vi "Escape_URL_method.vi"(8 "error in (no error)":errorcluster, 10 "Escape URLs?":bool, 11 "URL In":string) -> (0 "error out":errorcluster, 3 "URL Out":string)   [LabVIEW 2016]
uses:
  <vilib>/wsapi/NI_WebServices.lvlib
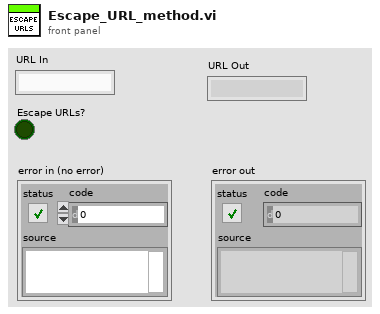
[diagram p1: front panel]
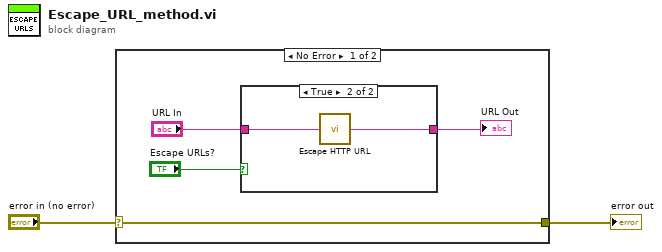
[diagram p0: block diagram]
diagram:
  n1 = case shown="No Error" "error in (no error)" {
    selector: "error in (no error)" -> [w3 w10]
    tunnel: [w3 w10] -> w1
    frame No Error {
      n2 = case shown="True" "Escape URLs?" {
        tunnel: "URL In" -> [w7 w9]
        tunnel: [w7 w8] -> w4
        frame False {
        }
        frame True {
          n3 = call <vilib>:"Escape HTTP URL.vi"("unescaped string in"=w9) -> ("escaped string out"=w8:string)
        }
      }
      "URL Out" <- w4
    }
    frame Error {
    }
  }
  "error out" <- w1
